vi "Remove_Trailing_Zero.vi"(1 "f":string) -> (0 "f 2":string)   [LabVIEW 2020]
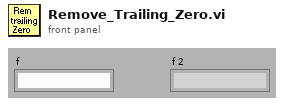
[diagram p1: front panel]
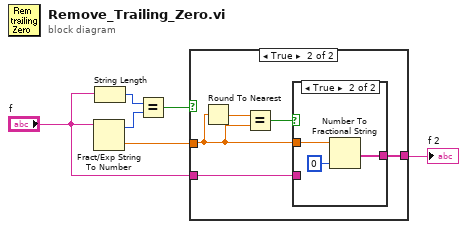
[diagram p0: block diagram]
diagram:
  n1 = Fract/Exp String To Number(string="f") -> (offset past number=w1:i32, number=w4:dbl)  [unwired: 3 out]
  n2 = String Length(string="f") -> (length=w2:i32)
  n3 = Equal?(x=w2, y=w1) -> (x = y?=w3:bool)
  n4 = case shown="True" w3 {
    tunnel: w4 -> [_ w10]
    tunnel: [w7 w9] -> w5
    tunnel: "f" -> [w7 w8]
    frame False {
    }
    frame True {
      n5 = Round To Nearest(number=w10) -> (nearest integer value=w12:dbl)
      n6 = Equal?(x=w12, y=w10) -> (x = y?=w11:bool)
      n7 = case shown="True" w11 {
        tunnel: w10 -> [_ w16]
        tunnel: [w13 w15] -> w9
        tunnel: w8 -> [w13 _]
        frame False {
        }
        frame True {
          n8 = Number To Fractional String(number=w16, precision (6)=i16 0) -> (F-format string=w15:string)  [unwired: 2 out]
        }
      }
    }
  }
  "f 2" <- w5
